vi "Test Parse U64 Space Delimited Array Ignoring Header.vi"(8 "error in (no error)":errorcluster, 11 "Test Case In":refnum<class "Helpers Test.lvclass">) -> (0 "error out":errorcluster, 3 "Test Case Out":refnum<class "Helpers Test.lvclass">)   [LabVIEW 2020, in "Helpers Test.lvclass"]
uses:
  Helpers Test.lvclass
  4993e8ee-a06a-463a-9684-69129f64d5ce.vi
  Helpers.lvlib
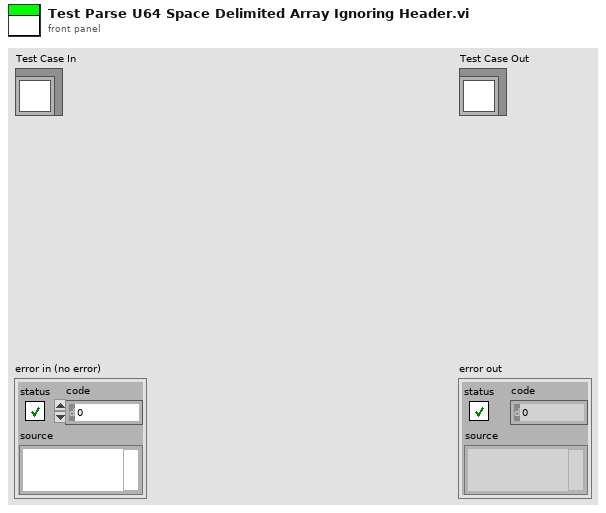
[diagram p1: front panel]
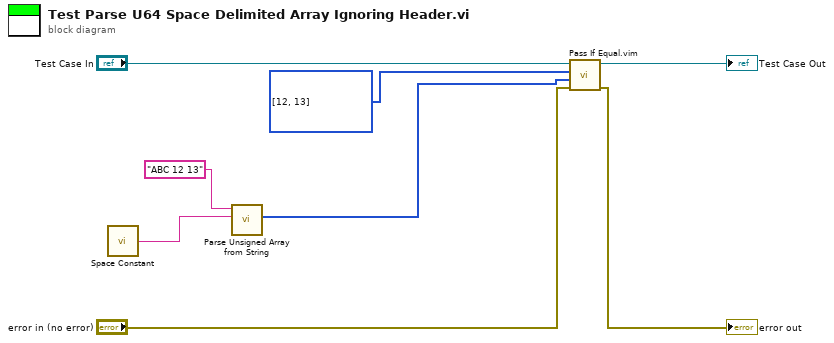
[diagram p0: block diagram]
diagram:
  n1 = call <vilib>:"Space Constant.vi"() -> ("String"=w3:string)
  n2 = call "Parse Unsigned Array from String.vi"("Delimiter regex"=w3, "Input"="ABC 12 13") -> ("Parsed U64 Array"=w1:u64[])  [unwired: 8 in, 1 out]
  n3 = call "Pass If Equal.vim"("error in (no error)"="error in (no error)", "Actual"=w1, "Expected"=u64[] [12, 13] ("Parsed Array"), "LUnit Test Case In"="Test Case In") -> ("error out"=→"error out":errorcluster, "LUnit Test Case Out"=→"Test Case Out":refnum<class "Helpers Test.lvclass">)  [unwired: 6 in]
